vi "GE 5565PIORC.PXI Interrupts.Wait for Event.vi"(8 "error in (no error)":errorcluster, 10 "timeout ms (1000)":u32=1000, 11 "GE 5565PIORC in":refnum<class "GE 5565PIORC.lvclass">) -> (0 "error out":errorcluster, 2 "timed out?":bool, 3 "GE 5565PIORC out":refnum<class "GE 5565PIORC.lvclass">)   [LabVIEW 2020, in "GE 5565PIORC.lvclass"]
doc: "Waits for an event to occur on PXI Interrupts for the GE 5565PIORC."
uses:
  GE 5565PIORC.lvclass
  GE 5565PIORC.lvclass/GE 5565PIORC.ctl
  <vilib>/Instr/_visa.llb/Select Event Type.ctl
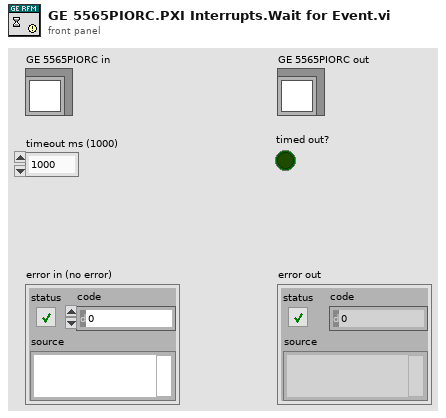
[diagram p1: front panel]
types:
  T1 = typedef "Select Event Type.ctl" = u32
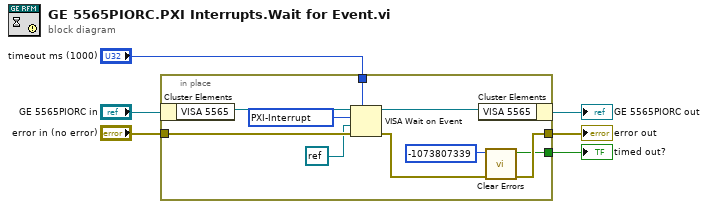
[diagram p0: block diagram]
diagram:
  n1 = in-place {
    in-place-border: "timeout ms (1000)" -> [w15]
    in-place-border: "error in (no error)" -> [w12]
    in-place-border: [w11] -> w5
    in-place-border: [w7] -> w4
    w16 = T1 1073684514 items=["ServiceRequest"=1073684491, "Trigger"=3221168138, "Clear"=1073684493, "VXI-Signal"=1073684512, "VXI/VME-Interrupt"=3221168161, "VXI/VME-Sysfail"=1073684509, "VXI/VME-Sysreset"=1073684510, "GPIB-CIC"=1073684498, "GPIB-Talk"=1073684499, "GPIB-Listen"=1073684500, "PXI-Interrupt"=1073684514, "AllEnabled"=1073709055] ("Event Type")
    n2 = in-place-cluster #1("GE 5565PIORC in") -> ("VISA 5565"=w9:refnum<visa-resource-name>)
    n3 = VISA Wait on Event(7:w15, 8:w12, 9:refnum<visa-resource-name> refnum ("event class (Generic Event)"), 10:w16, 11:w9) -> (0:w13:errorcluster, 3:w8:refnum<visa-resource-name>)  [unwired: 2 out]
    n4 = in-place-cluster #1("VISA 5565"=w8) -> (→"GE 5565PIORC out":refnum<class "GE 5565PIORC.lvclass">)
    n5 = call <vilib>:"Clear Errors.vi"("error in (no error)"=w13, "specific error code to clear (0: all)"=-1073807339) -> ("error out"=w11:errorcluster, "specific error cleared?"=w7:bool)  [unwired: 4 in]
  }
  "error out" <- w5
  "timed out?" <- w4
